vi "GenerateTDMSFile.vi"(0 "Directory":path, 1 "All Accelerometers?":bool, 5 "DeviceName":string="simRIO99", 7 "Number of Channels (per cRIO)":i32=18, 9 "Number Of Seconds":i32=1) -> (4 "Filepath":path, 15 "ErrorOut":errorcluster)   [LabVIEW 2017]
uses:
  <vilib>/addons/InsightCM/MessageBus/Base/controls/Device.ctl
  <vilib>/addons/InsightCM/MessageBus/Base/controls/KeyValuePair.ctl
  <vilib>/addons/InsightCM/MessageBus/Base/controls/DeviceState.ctl
  <vilib>/addons/InsightCM/MessageBus/Base/controls/DataGroup.ctl
  <vilib>/addons/InsightCM/MessageBus/Base/controls/BurstModeTrigger.ctl
  <vilib>/addons/InsightCM/MessageBus/Base/controls/Trigger.ctl
  <vilib>/addons/InsightCM/MessageBus/Base/controls/Condition.ctl
  <vilib>/addons/InsightCM/Utilities/TDMSFileGenerator/controls/Hierarchy_All.ctl
  <vilib>/addons/InsightCM/Utilities/TDMSFileGenerator/controls/Hierarchy_Line.ctl
  <vilib>/addons/InsightCM/Utilities/TDMSFileGenerator/controls/Hierarchy_Equipment.ctl
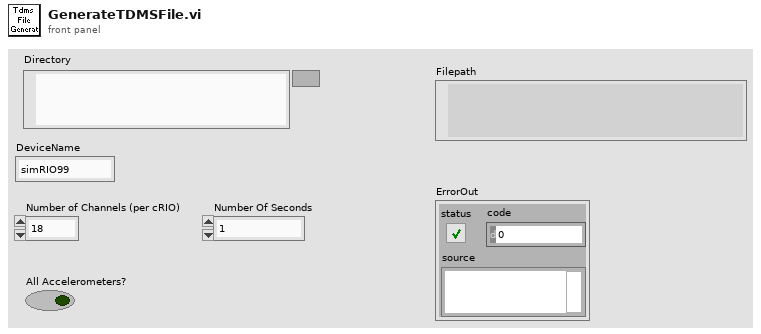
[diagram p1: front panel]
types:
  T1 = cluster{"1x":dbl, "2x":dbl, "3x":dbl, "8.5x":dbl, "30x":dbl}
  T2 = typedef "Hierarchy_Equipment.ctl" = cluster{"Equipment":string, "Components":string[]}
  T3 = typedef "Hierarchy_Line.ctl" = cluster{"Line":string, "Equipment":T2[]}
  T4 = typedef "Hierarchy_All.ctl" = cluster{"Enterprise":string, "Site":string, "Area":string, "Lines":T3[]}
  T5 = typedef "Device.ctl" = cluster{"Id":string, "Name":string, "DeviceType":string, "HardwareName":string, "IpAddress":string, "HardwareInfo":T6[], "ApplicationType":string, "ApplicationVersion":string, "ConfigurationVersion":string, "State":T7, "Properties":T6[], "DataGroups":T8[], "BurstModeTrigger":T9}
  T6 = typedef "KeyValuePair.ctl" = cluster{"Key":string, "Value":string}
  T7 = typedef "DeviceState.ctl" = cluster{"Disabled":bool}
  T8 = typedef "DataGroup.ctl" = cluster{"Name":string, "AssetNodeId":string}
  T9 = typedef "BurstModeTrigger.ctl" = cluster{"Trigger":T10, "SampleRate":string, "AcquisitionLength":string}
  T10 = typedef "Trigger.ctl" = cluster{"Type":string, "Expression":string, "Conditions":T11[]}
  T11 = typedef "Condition.ctl" = cluster{"Source":string, "Type":string, "Operator":string, "CompareTo":string, "DwellSeconds":dbl}
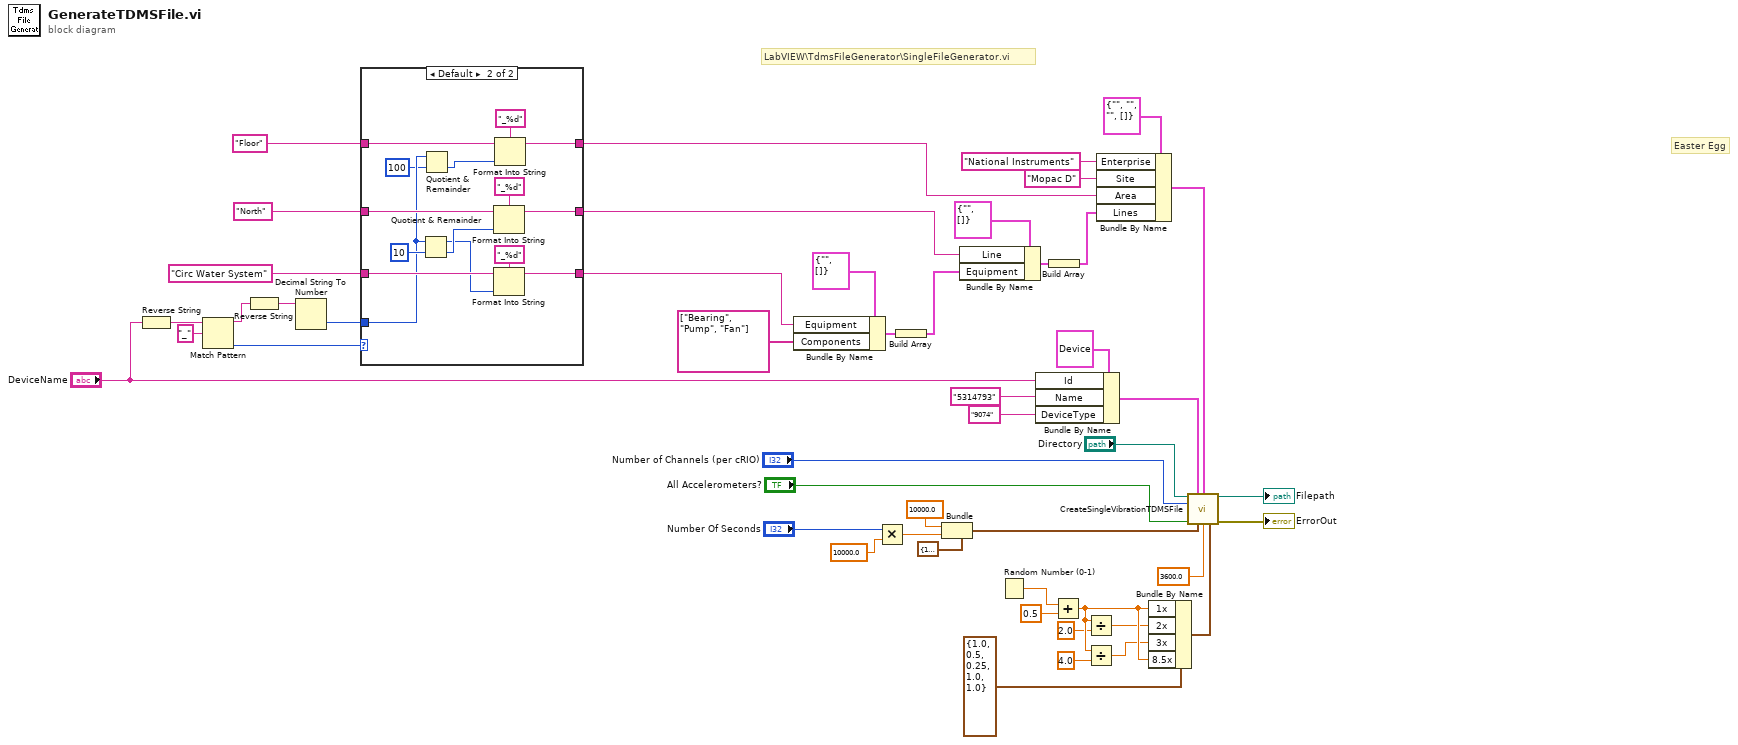
[diagram p0: block diagram]
diagram:
  # "Easter Egg"
  # "LabVIEW\\TdmsFileGenerator\\SingleFileGenerator.vi"
  n1 = Reverse String(1:"DeviceName") -> (0:w10:string)
  n2 = Match Pattern(string=w10, regular expression="_") -> (before substring=w8:string, offset past match=w2:i32)  [unwired: 1 in, 2 out]
  n3 = Reverse String(1:w8) -> (0:w7:string)
  n4 = Decimal String To Number(string=w7) -> (number=w4:i32)  [unwired: 2 in, 1 out]
  n5 = case shown="Default" w2 {
    tunnel: [w51 w65] -> w28
    tunnel: [w52 w61] -> w25
    tunnel: "North" ("Line") -> [w52 w62]
    tunnel: "Circ Water System" ("Equipment") -> [w51 w66]
    tunnel: w4 -> [_ w60]
    tunnel: "Floor" ("Area") -> [w50 w57]
    tunnel: [w50 w53] -> w1
    frame -1 {
    }
    frame Default {
      n6 = Quotient & Remainder(x=w60, y=10) -> (x-y*floor(x/y)=w54:i32, floor(x/y)=w55:i32)
      n7 = Quotient & Remainder(x=w60, y=100) -> (floor(x/y)=w56:i32)  [unwired: 1 out]
      n8 = Format Into String(format string="_%d", initial string=w62, w55) -> (resulting string=w61:string)  [unwired: 1 in, 1 out]
      n9 = Format Into String(format string="_%d", initial string=w66, w54) -> (resulting string=w65:string)  [unwired: 1 in, 1 out]
      n10 = Format Into String(format string="_%d", initial string=w57, w56) -> (resulting string=w53:string)  [unwired: 1 in, 1 out]
    }
  }
  n11 = Bundle By Name(cluster=T2 {"Equipment"="", "Components"=[]} ("Equipment"), "Equipment"=w28, "Components"=string[] ["Bearing", "Pump", "Fan"]) -> (w27:T2)
  n12 = Multiply(x="Number Of Seconds", y=10000.0 ("Fs")) -> (x*y=w14:dbl)
  n13 = Build Array(w27) -> (w26:T2[])
  n14 = Bundle(cluster=cluster{"Fs":dbl, "#s":dbl} {"Fs"=10000.0, "#s"=100000.0} ("sampling info"), "Fs"=10000.0, "#s"=w14) -> (w40:cluster{"Fs":dbl, "#s":dbl})
  n15 = Bundle By Name(cluster=T3 {"Line"="", "Equipment"=[]} ("Line"), "Line"=w25, "Equipment"=w26) -> (w24:T3)
  n16 = Random Number (0-1)() -> (number: 0 to 1=w47:dbl)
  n17 = Bundle By Name(cluster=T5 {"Id"="", "Name"="", "DeviceType"="", "HardwareName"="", "IpAddress"="", "HardwareInfo"=[], "ApplicationType"="", "ApplicationVersion"="", "ConfigurationVersion"="", "State"={"Disabled"=FALSE}, "Properties"=[], "DataGroups"=[], "BurstModeTrigger"={"Trigger"={"Type"="", "Expression"="", "Conditions"=[]}, "SampleRate"="", "AcquisitionLength"=""}} ("Device"), "Id"="DeviceName", "Name"="5314793" ("Device Serial Number"), "DeviceType"="9074" ("Device Model")) -> (w34:T5)
  n18 = Build Array(w24) -> (w23:T3[])
  n19 = Add(x=w47, y=0.5) -> (x+y=w45:dbl)
  n20 = Divide(x=w45, y=2.0) -> (x/y=w42:dbl)
  n21 = Divide(x=w45, y=4.0) -> (x/y=w41:dbl)
  n22 = Bundle By Name(cluster=T4 {"Enterprise"="", "Site"="", "Area"="", "Lines"=[]} ("Hierarchy"), "Enterprise"="National Instruments", "Site"="Mopac D", "Area"=w1, "Lines"=w23) -> (w22:T4)
  n23 = Bundle By Name(cluster=T1 {"1x"=1.0, "2x"=0.5, "3x"=0.25, "8.5x"=1.0, "30x"=1.0} ("Amplitude"), "1x"=w45, "2x"=w42, "3x"=w41, "8.5x"=w45) -> (w17:T1)
  n24 = call <vilib>:"CreateSingleVibrationTDMSFile.vi"("Requested Directory"="Directory", "Device"=w34, "Hierarchy"=w22, "Number of Channels"="Number of Channels (per cRIO)", "All Accelerometers?"="All Accelerometers?", "sampling info"=w40, "Running Speed (RPM)"=3600.0, "Amplitude"=w17) -> ("Created File"=→"Filepath":path, "error out"=→"ErrorOut":errorcluster)  [unwired: 6 in]
